vi "CheatGlobals.vi"() -> ()   [LabVIEW 2019]
panel:
  out "DiscoMode":bool
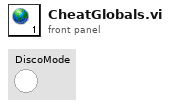
[diagram p1: front panel]
diagram:
